vi "BR ACT manual cmd (SubVI).vi"(4 "freq":dbl=1.0 format="%#_13g", 5 "Array of Double in":dbl[](array[numeric]), 6 "amp":dbl=8.0 format="%#_13g", 7 "BR ACT - Manual cmd":bool, 8 "BR ACT - Manual cmd osc p":bool, 9 "BR ACT - Manual cmd osc y":bool, 10 "Atuador Pitch [Deg]":dbl(knob) scale=-4.0..4.0, 11 "Atuador Yaw [Deg]":dbl(knob) scale=-4.0..4.0) -> (3 "Array of Double out":dbl[](array[numeric]))   [LabVIEW 2017]
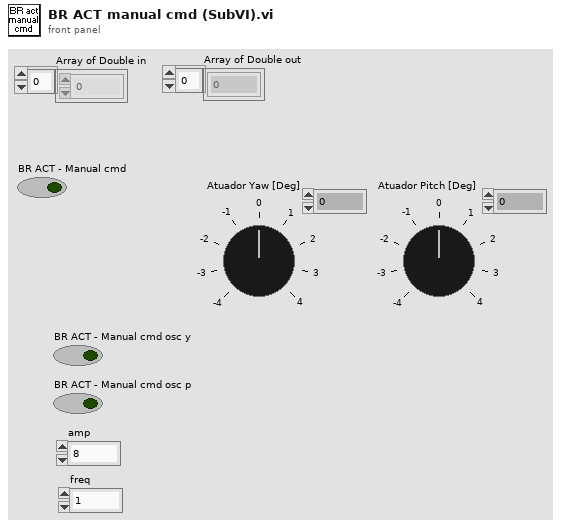
[diagram p1: front panel]
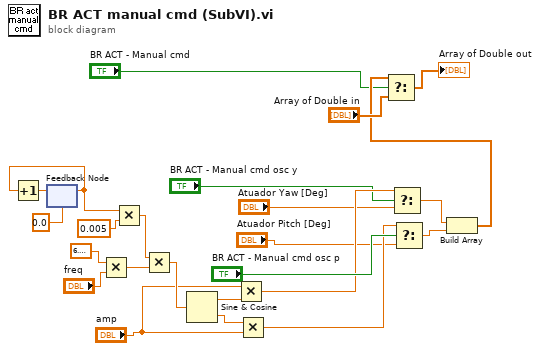
[diagram p0: block diagram]
diagram:
  n1 = feedback #1(0.0) -> (w13:dbl)
  n2 = Increment(x=w13) -> (x+1=w12:dbl)
  n3 = feedback-in #1(w12) -> ()
  n4 = Multiply(x=6.283185307179586, y="freq") -> (x*y=w11:dbl)
  n5 = Multiply(x=w13, y=0.005) -> (x*y=w15:dbl)
  n6 = Multiply(x=w15, y=w11) -> (x*y=w16:dbl)
  n7 = Sine & Cosine(0:w16) -> (1:w6:dbl, 2:w8:dbl)
  n8 = Multiply(x="amp", y=w6) -> (x*y=w22:dbl)
  n9 = Multiply(x=w8, y="amp") -> (x*y=w23:dbl)
  n10 = Select(t=w22, s="BR ACT - Manual cmd osc y", f="Atuador Yaw [Deg]") -> (s? t:f=w21:dbl)
  n11 = Select(t=w23, s="BR ACT - Manual cmd osc p", f="Atuador Pitch [Deg]") -> (s? t:f=w20:dbl)
  n12 = Build Array(w21, w20) -> (w2:dbl[])
  n13 = Select(t=w2, s="BR ACT - Manual cmd", f="Array of Double in") -> (s? t:f=→"Array of Double out":dbl[])
